vi "SampleAvg.Generate Accumulator DataValids (prefetch).vi"(8 "Input Valid":bool=TRUE, 9 "New Record?":bool=TRUE, 10 "Load New Count":bool=TRUE, 11 "Count":i16) -> (0 "Output Valid":bool=TRUE, 1 "New Record":bool=TRUE, 2 "NewCount?":bool, 3 "Count":i16, 4 "WasInputValid?":bool=TRUE, 6 "Get New Load":bool)   [LabVIEW 2014]
doc: "<b> Latency = 1 Tick </b>"
panel:
  # "Copyright 2014 Vidrio Technologies\nScanImage 5 software is licensed under the Apache License, Version 2.0 (the \"License\"); you may not use any files contained\nwithin the ScanImage 5 release except in compliance with the License. You may obtain a copy of the License at\n http://www.apache.org/licenses/LICENSE-2.0\nUnless required by applicable law or agreed to in writing, software distributed under the License is distributed on an\n\"AS IS\" BASIS, WITHOUT WARRANTIES OR CONDITIONS OF ANY KIND, either express or implied. See the License for the\n specific language governing permissions and limitations under the License."
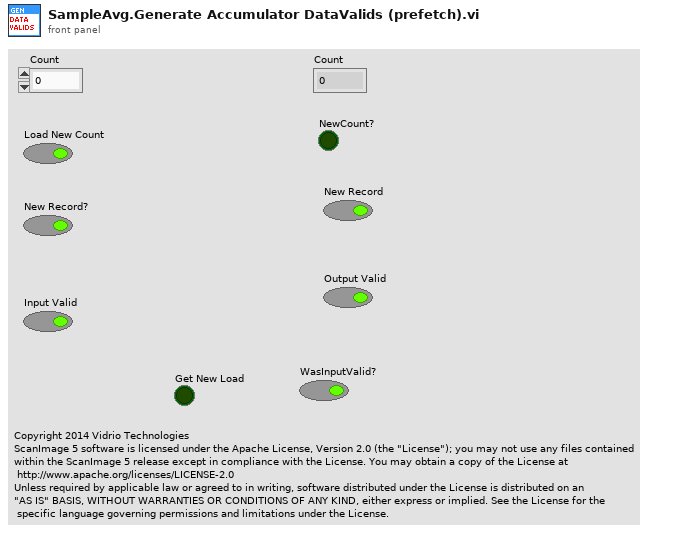
[diagram p1: front panel]
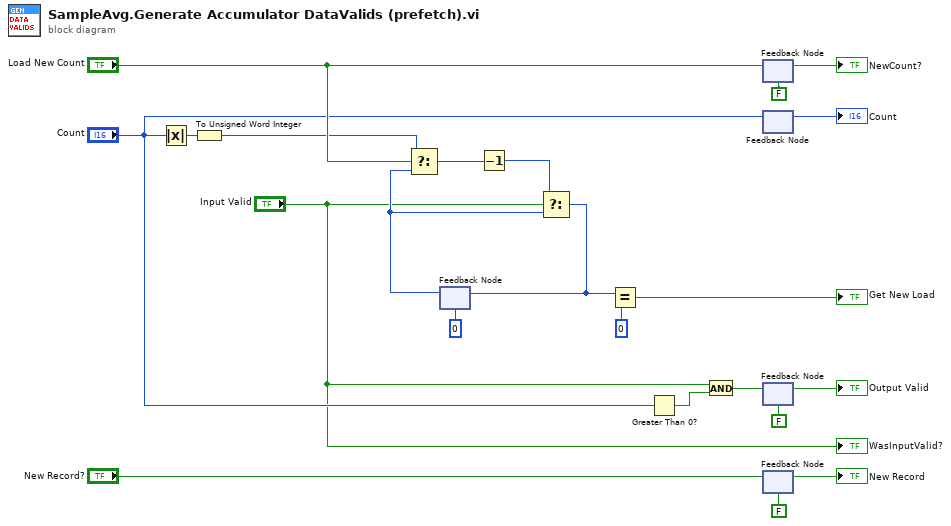
[diagram p0: block diagram]
diagram:
  n1 = Absolute Value(x="Count") -> (abs(x)=w4:i16)
  n2 = To Unsigned Word Integer(number=w4) -> (unsigned 16bit integer=w7:u16)
  n3 = feedback #1(u16 0) -> (w15:u16)
  n4 = Select(t=w7, s="Load New Count", f=w15) -> (s? t:f=w21:u16)
  n5 = Decrement(x=w21) -> (x-1=w16:u16)
  n6 = Select(t=w16, s="Input Valid", f=w15) -> (s? t:f=w14:u16)
  n7 = feedback-in #1(w14) -> ()
  n8 = Equal?(x=w14, y=u16 0) -> (x = y?=→"Get New Load":bool)
  n9 = Greater Than 0?(x="Count") -> (x > 0?=w5:bool)
  n10 = And(x="Input Valid", y=w5) -> (x .and. y?=w6:bool)
  n11 = feedback #2(FALSE) -> (→"NewCount?":bool)
  n12 = feedback-in #2("Load New Count") -> ()
  n13 = feedback-in #3("Count") -> ()
  n14 = feedback #3() -> (→"Count":i16)  [unwired: 1 in]
  n15 = feedback #4(FALSE ("Input Valid")) -> (→"Output Valid":bool)
  n16 = feedback-in #4(w6) -> ()
  n17 = feedback #5(FALSE) -> (→"New Record":bool)
  n18 = feedback-in #5("New Record?") -> ()
  "WasInputValid?" <- "Input Valid"
